vi "deCOB-ID.vi"(0 "Cob ID":u32 format="%.0x") -> (1 "Node ID":u8, 2 "Function code":T1 items=["EMCY"=1, "PDO1 (tx)"=3, "PDO1 (rx)"=4, "PDO2 (tx)"=5, "PDO2 (rx)"=6, "PDO3 (tx)"=7, "PDO3 (rx)"=8, "PDO4 (tx)"=9, "PDO4 (rx)"=10, "SDO (tx)"=11, "SDO (rx)"=12, "NMT error control"=14])   [LabVIEW 2026, in "canopen_.lvlib" / "CANopen.lvclass"]
doc: "Decomposes a canonical COB-ID into its function code and node ID. This is the reverse operation of enCOB-ID."
uses:
  CANopen.lvclass
  CANopen.lvclass/CANopen.ctl
  FunctionCode.ctl
  CANopen Master.lvlib
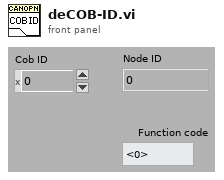
[diagram p1: front panel]
types:
  T1 = typedef "CANopen Master.lvlib/FunctionCode.ctl" = u16
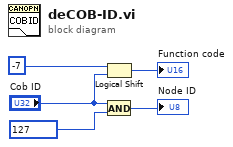
[diagram p0: block diagram]
diagram:
  n1 = Logical Shift(y=i16 -7, x="Cob ID") -> (x << y=→"Function code":u32)
  n2 = And(x="Cob ID", y=u32 127) -> (x .and. y?=→"Node ID":u32)
